vi "Main_flow.vi"() -> ()   [LabVIEW 2022 SP3]
panel:
  in  "temp":dbl
  in  "Hand DOWN":bool
  in  "Hand UP":bool
  in  "Trigger Period(sec)":dbl
  out "Current Time":dbl
  in  "Counter":dbl
  out "Buzzer":bool
  in  "Man Entered":bool
  in  "Mode":dbl
  in  "stop":bool
  in  "Capacitor Detected":bool
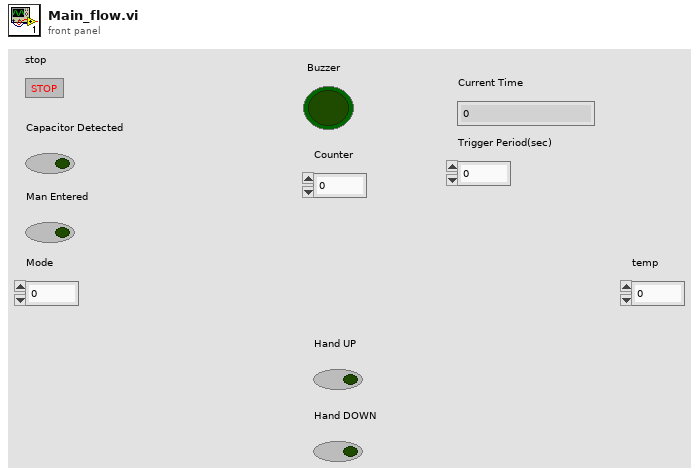
[diagram p1: front panel]
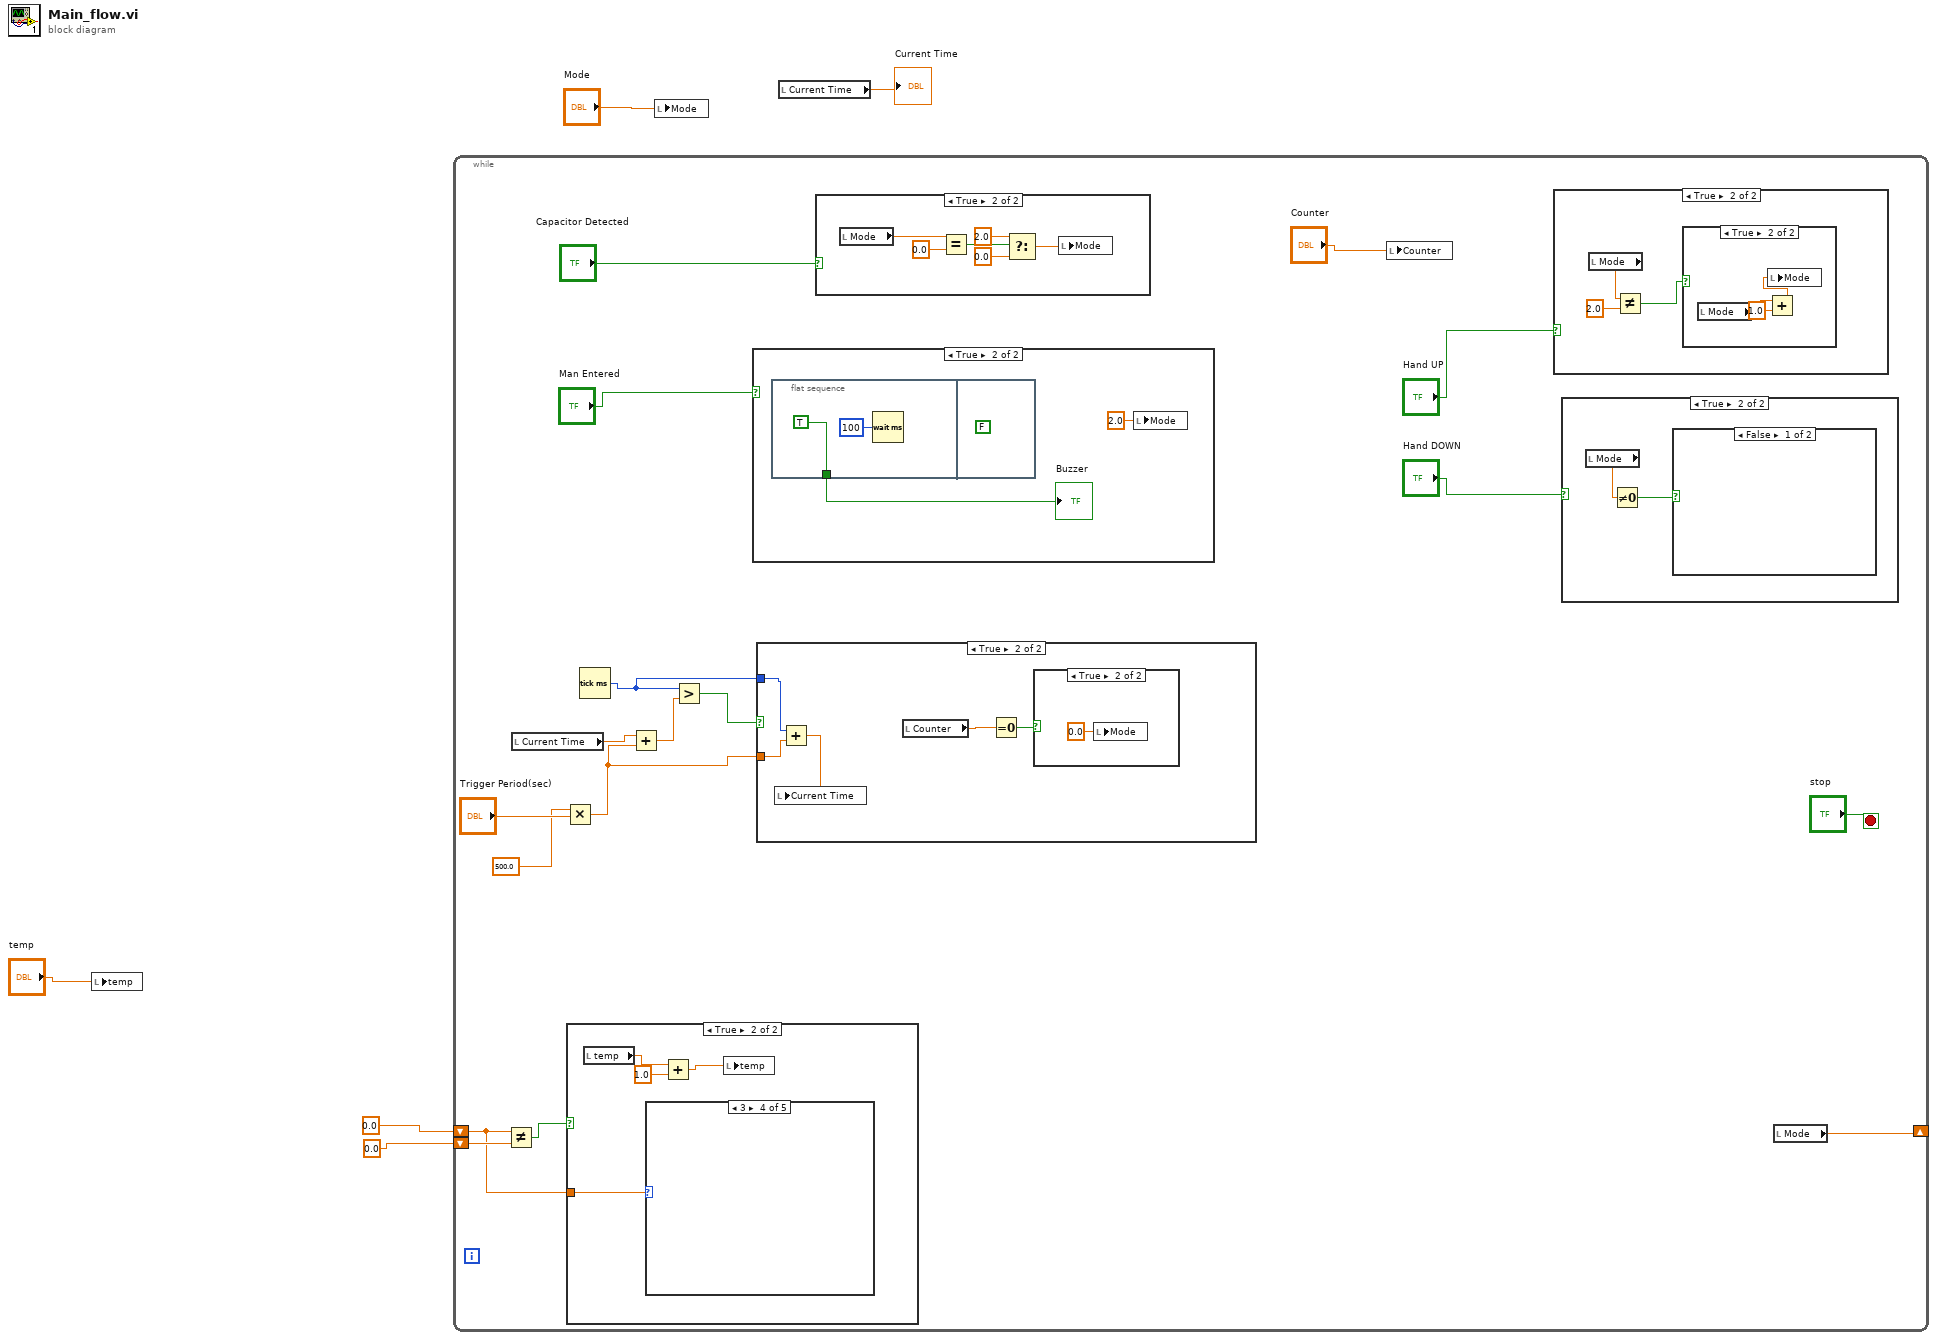
[diagram p0: block diagram]
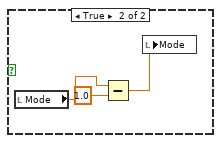
[diagram p8: hidden frame]
diagram:
  n1 = local write "temp"("temp") -> ()
  n2 = while {
    shift-right: [w9] -> _
    shift-left: 0.0 ("Mode") -> [w6]
    shift-left: 0.0 ("Mode") -> [w8]
    stop <- "stop" stop-if-true
    n3 = Not Equal?(x=w6, y=w8) -> (x != y?=w7:bool)
    n4 = local read "Current Time"() -> (w18:dbl)
    n5 = Multiply(x=500.0, y="Trigger Period(sec)") -> (x*y=w12:dbl)
    n6 = case shown="True" w7 {
      tunnel: w6 -> [_ w23]
      frame False {
      }
      frame True {
        n7 = local read "temp"() -> (w26:dbl)
        n8 = case shown="3" w23 {
          frame 0 {
          }
          frame 1 {
          }
          frame 2 {
          }
          frame 3 {
          }
          frame Default {
          }
        }
        n9 = Add(x=w26, y=1.0) -> (x+y=w25:dbl)
        n10 = local write "temp"(w25) -> ()
      }
    }
    n11 = Tick Count (ms)() -> (millisecond timer value=w16:u32)
    n12 = Add(x=w18, y=w12) -> (x+y=w15:dbl)
    n13 = Greater?(x=w16, y=w15) -> (0:w17:bool)
    n14 = case shown="True" "Man Entered" {
      frame False {
      }
      frame True {
        n15 = flat-sequence {
          tunnel: [TRUE] -> w45
          frame #0 {
            n16 = Wait (ms)(milliseconds to wait=u32 100) -> ()  [unwired: 1 out]
          }
          frame #1 {
            (unwired) FALSE
          }
        }
        n17 = local write "Mode"(2.0 ("Mode")) -> ()
        "Buzzer" <- w45
      }
    }
    n18 = case shown="True" w17 {
      tunnel: w16 -> [_ w41]
      tunnel: w12 -> [_ w40]
      frame False {
      }
      frame True {
        n19 = Add(x=w41, y=w40) -> (x+y=w42:dbl)
        n20 = local write "Current Time"(w42) -> ()
        n21 = local read "Counter"() -> (w39:dbl)
        n22 = Equal To 0?(x=w39) -> (x = 0?=w38:bool)
        n23 = case shown="True" w38 {
          frame False {
          }
          frame True {
            n24 = local write "Mode"(0.0 ("Mode")) -> ()
          }
        }
      }
    }
    n25 = case shown="True" "Capacitor Detected" {
      frame False {
      }
      frame True {
        n26 = local read "Mode"() -> (w53:dbl)
        n27 = Equal?(x=w53, y=0.0) -> (x = y?=w51:bool)
        n28 = Select(t=2.0, s=w51, f=0.0) -> (s? t:f=w50:dbl)
        n29 = local write "Mode"(w50) -> ()
      }
    }
    n30 = local write "Counter"("Counter") -> ()
    n31 = case shown="True" "Hand UP" {
      frame False {
      }
      frame True {
        n32 = local read "Mode"() -> (w34:dbl)
        n33 = Not Equal?(x=w34, y=2.0) -> (x != y?=w32:bool)
        n34 = case shown="True" w32 {
          frame False {
          }
          frame True {
            n35 = local read "Mode"() -> (w37:dbl)
            n36 = Add(x=w37, y=1.0) -> (x+y=w35:dbl)
            n37 = local write "Mode"(w35) -> ()
          }
        }
      }
    }
    n38 = case shown="True" "Hand DOWN" {
      frame False {
      }
      frame True {
        n39 = local read "Mode"() -> (w28:dbl)
        n40 = Not Equal To 0?(x=w28) -> (x != 0?=w27:bool)
        n41 = case shown="False" w27 {
          frame False {
          }
          frame True {
            n42 = local read "Mode"() -> (w30:dbl)
            n43 = Subtract(x=w30, y=1.0) -> (x-y=w29:dbl)
            n44 = local write "Mode"(w29) -> ()
          }
        }
      }
    }
    n45 = local read "Mode"() -> (w9:dbl)
  }
  n46 = local write "Mode"("Mode") -> ()
  n47 = local read "Current Time"() -> (→"Current Time":dbl)
